vi "Wait_seconds.vi"(0 "Seconds to wait":u32) -> ()   [LabVIEW 2010]
panel:
  out "No of seconds waited":u32
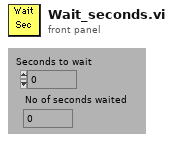
[diagram p1: front panel]
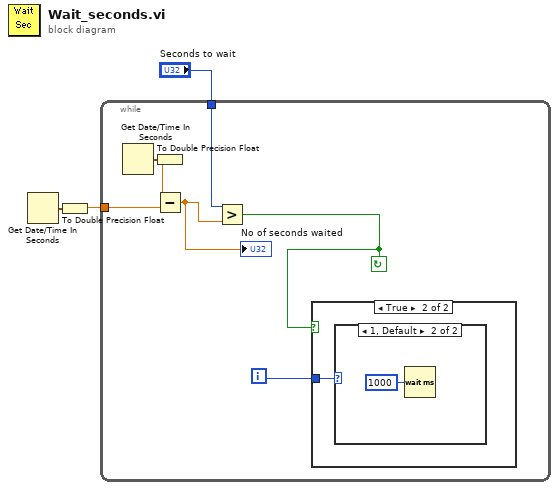
[diagram p0: block diagram]
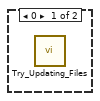
[diagram p3: hidden frame]
diagram:
  n1 = Get Date/Time In Seconds() -> (seconds since 1Jan1904=w1:timestamp)
  n2 = To Double Precision Float(number=w1) -> (double precision float=w2:dbl)
  n3 = while {
    tunnel: "Seconds to wait" -> [w9]
    tunnel: w2 -> [w10]
    i -> [w4]
    stop <- w5 continue-if-true
    n4 = Get Date/Time In Seconds() -> (seconds since 1Jan1904=w6:timestamp)
    n5 = To Double Precision Float(number=w6) -> (double precision float=w7:dbl)
    n6 = Subtract(x=w7, y=w10) -> (x-y=w8:dbl)
    "No of seconds waited" <- w8
    n7 = Greater?(x=w9, y=w8) -> (0:w5:bool)
    n8 = case shown="True" w5 {
      tunnel: w4 -> [_ w11]
      frame False {
      }
      frame True {
        n9 = case shown="1, Default" w11 {
          frame 0 {
            n10 = call "Try_Updating_Files.vi"() -> ()  [unwired: 4 out]
          }
          frame 1, Default {
            n11 = Wait (ms)(milliseconds to wait=u32 1000) -> ()  [unwired: 1 out]
          }
        }
      }
    }
  }
